vi "Build--function.vi"(5 "Wait for debugger on launch (false)":bool, 6 "VersionString":string="v0.4.0-rc2_htr404testing", 7 "Enable debugging (false)":bool, 8 "error in":errorcluster, 9 "DestinationDir":path=path "C:/Users/pauloneill/SCC/Orion/LabVIEW/Builds/Orion", 10 "BuildSpec":string="Orion", 11 "ProjectPath":path=path "C:/Users/pauloneill/SCC/Orion/LabVIEW/Source/App/Orion.lvproj") -> (0 "error out":errorcluster, 2 "GeneratedFiles":path[](array[path]))   [LabVIEW 2020, in "CICD.lvlib"]
doc: "Sets the build output folder before building the application. Run this VI using LabVIEW CLI with the input build spec name to set the output path relative to the git root."
uses:
  CICD.lvlib
  <vilib>/ErrorRing/Error Ring.xnode
  <vilib>/Utility/error.llb/Error Cluster From Error Code.vi
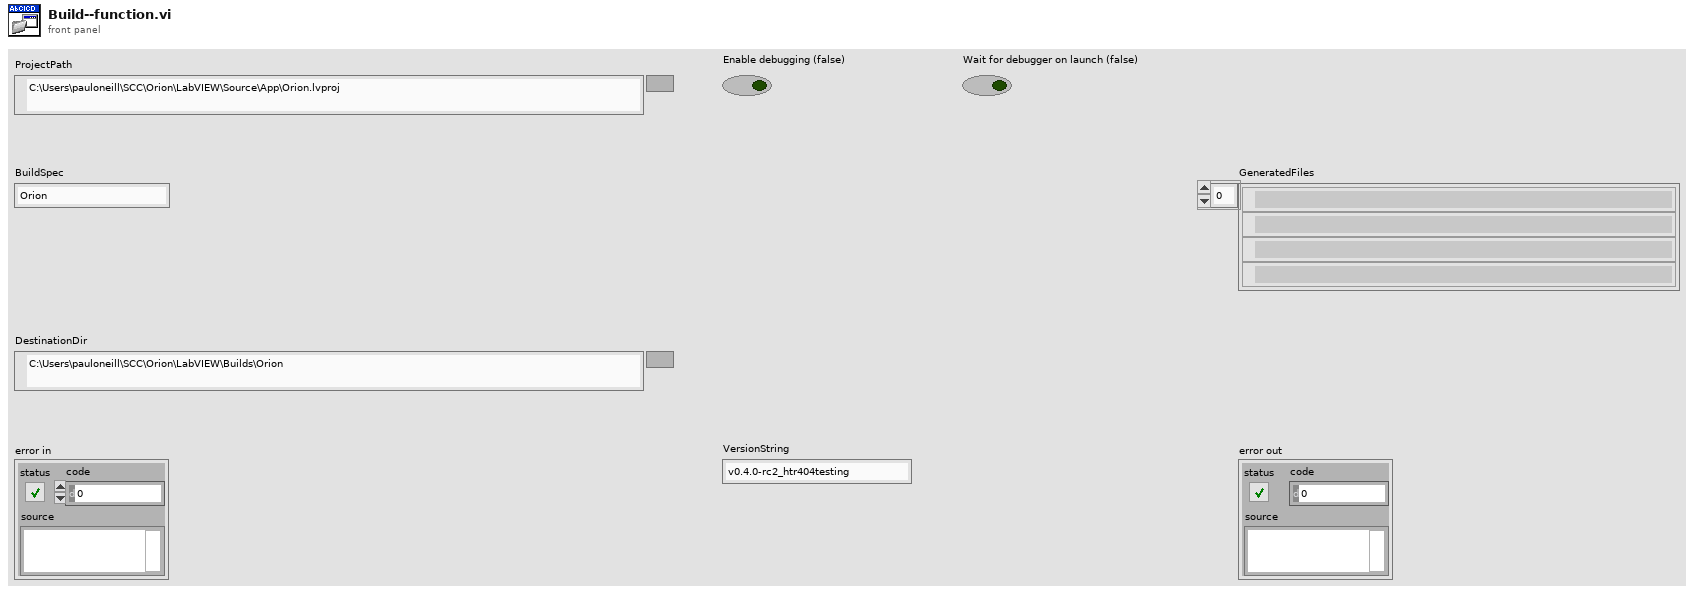
[diagram p1: front panel]
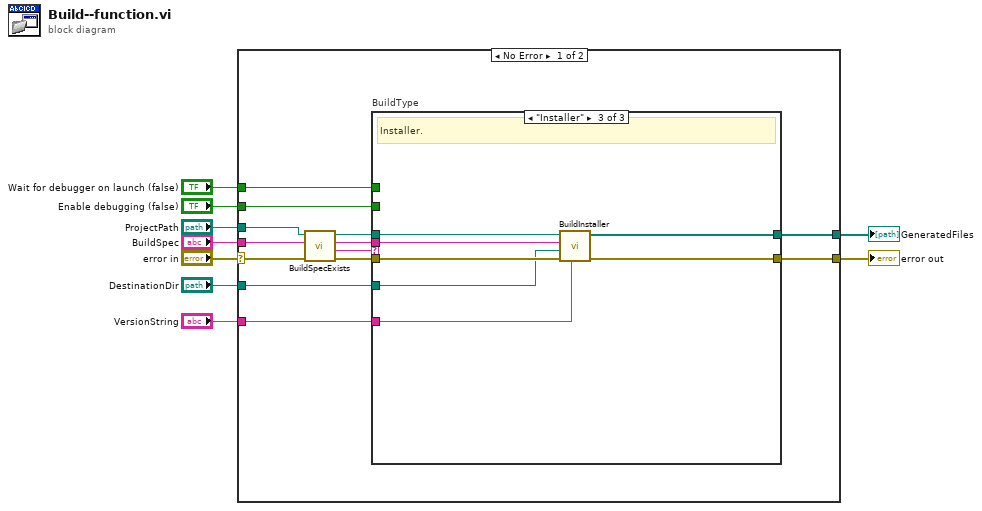
[diagram p0: block diagram]
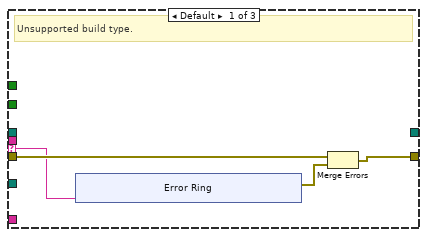
[diagram p2: hidden frame]
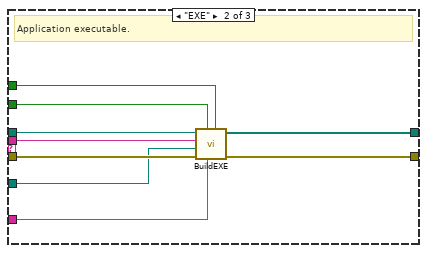
[diagram p3: hidden frame]
diagram:
  n1 = case shown="No Error" "error in" {
    selector: "error in" -> [w20 w50]
    tunnel: [w21 w50] -> w9
    tunnel: "ProjectPath" -> [w19 _]
    tunnel: "BuildSpec" -> [w18 _]
    tunnel: "DestinationDir" -> [w17 _]
    tunnel: [w16 _] -> w4
    tunnel: "VersionString" -> [w15 _]
    tunnel: "Enable debugging (false)" -> [w11 _]
    tunnel: "Wait for debugger on launch (false)" -> [w10 _]
    frame No Error {
      n2 = call "BuildSpecExists.vi"("error in"=w20, "BuildSpec in"=w18, "ProjectPath"=w19) -> ("error out"=w22:errorcluster, "Build Type"=w13:string, "BuildSpec out"=w12:string, "ProjectPath dup"=w14:path)  [unwired: 5 in]
      n3 = case "BuildType" shown="\"Installer\"" w13 {
        selector: w13 -> [w23 _ _]
        tunnel: w22 -> [w26 w42 w49]
        tunnel: [w25 w41 w48] -> w21
        tunnel: w17 -> [_ w40 w45]
        tunnel: [_ w39 w43] -> w16
        tunnel: w15 -> [_ w38 w44]
        tunnel: w14 -> [_ w37 w47]
        tunnel: w12 -> [_ w36 w46]
        tunnel: w11 -> [_ w35 _]
        tunnel: w10 -> [_ w34 _]
        frame Default {
          # "Unsupported build type."
          n4 = xnode "Error Ring"("parameter 0"=w23) -> ("error out"=w24:errorcluster)
          n5 = Merge Errors(w26, w24) -> (w25:errorcluster)
        }
        frame "EXE" {
          # "Application executable."
          n6 = call "BuildEXE.vi"("Wait for debugger on launch (false)"=w34, "VersionString"=w38, "Enable debugging (false)"=w35, "error in"=w42, "DestinationDir"=w40, "BuildSpec"=w36, "ProjectPath"=w37) -> ("error out"=w41:errorcluster, "GeneratedFiles"=w39:path[])  [unwired: 3 in]
        }
        frame "Installer" {
          # "Installer."
          n7 = call "BuildInstaller.vi"("VersionString"=w44, "error in"=w49, "DestinationDir"=w45, "BuildSpec"=w46, "ProjectPath"=w47) -> ("error out"=w48:errorcluster, "Generated files"=w43:path[])  [unwired: 5 in]
        }
      }
    }
    frame Error {
    }
  }
  "error out" <- w9
  "GeneratedFiles" <- w4
